vi "Start Logging.vi"(0 "reference in":refnum<class "Logger.lvclass">, 5 "file path":path, 7 "group name":string, 9 "channel name":string[](array[string]), 11 "Error In":errorcluster) -> (4 "reference out":refnum<class "Logger.lvclass">, 15 "Error Out":errorcluster)   [LabVIEW 2024, in "Logger.lvclass"]
uses:
  Logger.lvclass
panel:
  # "Connector Pane"
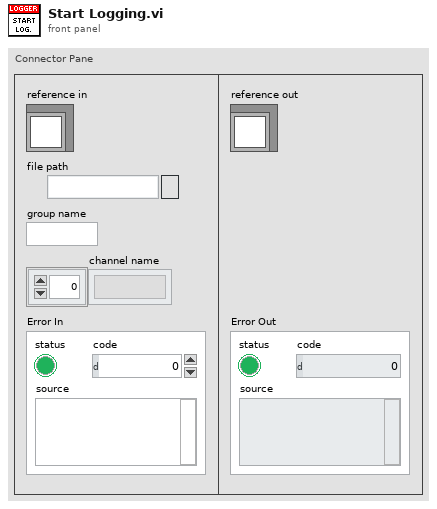
[diagram p1: front panel]
types:
  T1 = enum16{"open", "open or create", "create or replace", "create", "open (read-only)"}
  T2 = typedef "Logger.lvclass/ObjectAttributes.ctl" = cluster{"TDMS File":refnum<k34>, "Channel Names":string[], "Group Name":string}
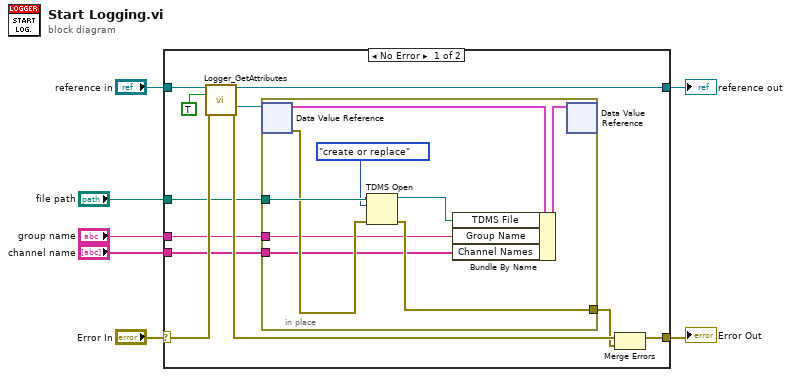
[diagram p0: block diagram]
diagram:
  n1 = case shown="No Error" "Error In" {
    selector: "Error In" -> [w17 w29]
    tunnel: [w15 w29] -> w6
    tunnel: [w16 w28] -> w4
    tunnel: "reference in" -> [w18 w28]
    tunnel: "file path" -> [w11 _]
    tunnel: "group name" -> [w10 _]
    tunnel: "channel name" -> [w9 _]
    frame No Error {
      n2 = call "Logger_GetAttributes.vi"("reference in"=w18, "OnlyGetDvrReference(False)"=TRUE, "Error In"=w17) -> ("reference out"=w16:refnum<class "Logger.lvclass">, "DataRef"=w14:refnum<data-value>, "Error Out"=w13:errorcluster)  [unwired: 9 in, 1 out]
      n3 = in-place {
        in-place-border: w11 -> [w25]
        in-place-border: w10 -> [w20]
        in-place-border: w9 -> [w19]
        in-place-border: [w23] -> w8
        n4 = in-place-dvr #1(w14) -> (w26:T2, w21:errorcluster)
        n5 = TDMS Open(8:w21, 10:T1."create or replace" ("operation (0:open)"), 11:w25) -> (0:w23:errorcluster, 3:w22:refnum<k34>)  [unwired: 4 in]
        n6 = Bundle By Name(cluster=w26, "TDMS File"=w22, "Group Name"=w20, "Channel Names"=w19) -> (w27:T2)
        n7 = in-place-dvr #1(w27) -> ()  [unwired: 2 out]
      }
      n8 = Merge Errors(w13, w8) -> (w15:errorcluster)
    }
    frame Error {
    }
  }
  "Error Out" <- w6
  "reference out" <- w4
